vi "TLC Main.vi"() -> ()   [LabVIEW 2009]
doc: "This VI is the Main VI of the Traffic Light Application. The Traffic Light Application is responsible for maintaining traffic at a heavily used 4-way intersection. The intersection includes North, South, East and West bound traffic, with each direction having a left-hand turn lane.\n\nSensors are present at each direction, and the left turn sequence is only inserted if a vehicle is positioned over the left turn lane sensor at the time the left turn sequence should start.\n\nSee the Requirement Document for the detailed pattern of no left-turn and left-turn sequences."
uses:
  controls/tlc_TrafficLightDisplay_cluster.ctl
  controls/tlc_TrafficLightLeftDisplay_cluster.ctl
  modules/controller/tlc_controller_SensorData_cluster.ctl
  controls/tlc_ConsumerDataType_enum.ctl
  controls/tlc_ConsumerCommand_enum.ctl
  modules/error/tlc_error_Command_enum.ctl
  modules/controller/tlc_controller_Command_enum.ctl
panel:
  out "error out":errorcluster
  in  "error in (no error)":errorcluster
  in  "Sensors (type)":T1
  in  "North Sensor":bool
  in  "West Sensor":bool
  in  "East Sensor":bool
  in  "South Sensor":bool
  in  "Stop":bool
  out "West Bound Left":T2
  out "West Bound":T3
  out "North Bound Left":T2
  out "North Bound":T3
  out "East Bound Left":T2
  out "East Bound":T3
  out "South Bound Left":T2
  out "South Bound":T3
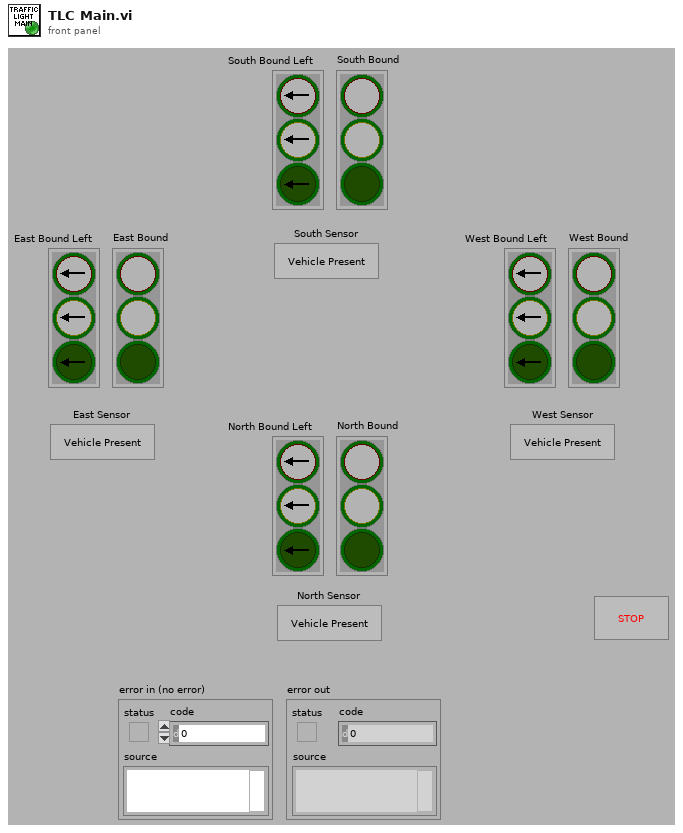
[diagram p1: front panel]
types:
  T1 = typedef "tlc_controller_SensorData_cluster.ctl" = cluster{"South Sensor":bool, "East Sensor":bool, "North Sensor":bool, "West Sensor":bool}
  T2 = typedef "tlc_TrafficLightLeftDisplay_cluster.ctl" = cluster{"Red":bool, "Yellow":bool, "Green":bool}
  T3 = typedef "tlc_TrafficLightDisplay_cluster.ctl" = cluster{"Red":bool, "Yellow":bool, "Green":bool}
  T4 = typedef "tlc_error_Command_enum.ctl" = enum16{"Initialise", "Check Error", "Report Errors"}
  T5 = typedef "tlc_ConsumerDataType_enum.ctl" = cluster{"Command":T6, "Data":variant}
  T6 = typedef "tlc_ConsumerCommand_enum.ctl" = enum16{"Initialise", "Check Controller", "Exit"}
  T7 = typedef "tlc_controller_Command_enum.ctl" = enum16{"Initialise", "Check State", "Next State Logic", "Set Traffic Lights", "Shutdown"}
  T8 = typedef "tlc_controller_TrafficLightsData_cluster.ctl" = cluster{"N/S":T3, "N/S Left":T2, "E/W":T3, "E/W Left":T2}
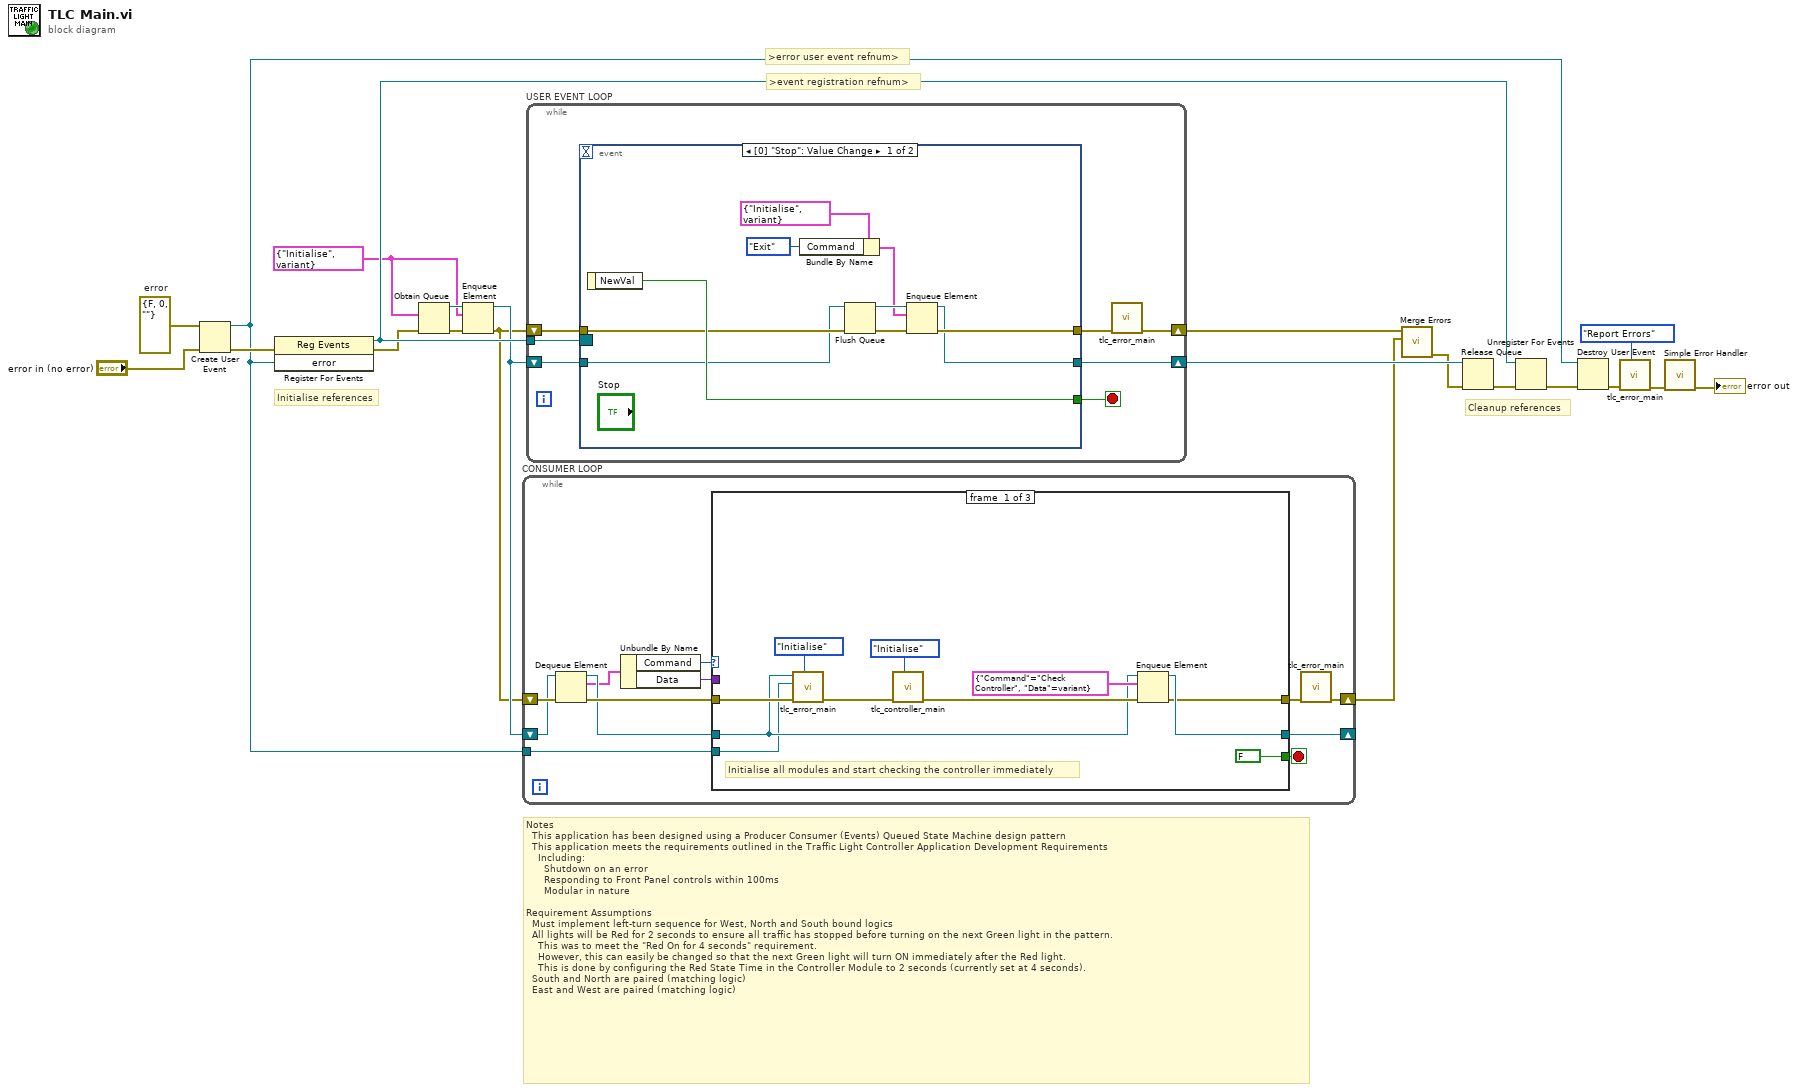
[diagram p0: block diagram]
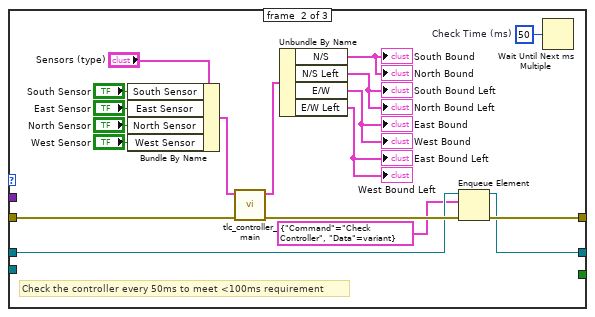
[diagram p2: hidden frame]
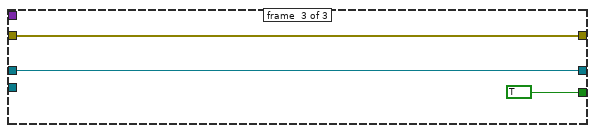
[diagram p3: hidden frame]
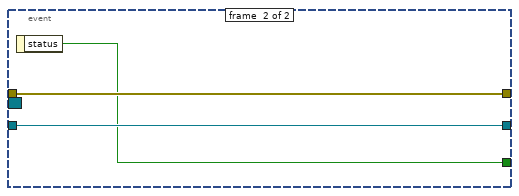
[diagram p4: hidden frame]
diagram:
  w14 = T5 {"Command"=enum."Initialise", "Data"=variant} ("Consumer Data Type")
  w21 = errorcluster {"status"=FALSE, "code"=0, "source"=""}  # error
  # "Notes\n  This application has been designed using a Producer Consumer (Events) Queued State Machine design pattern\n  This application meets the requirements outlined in the Traffic Light Controller Application Development Requirements\n    Including:\n      Shutdown on an error\n      Responding to Front Panel controls within 100ms\n      Modular in nature\n\nRequirement Assumptions\n  Must implement left-turn sequence for West, North and South bound logics\n  All lights will be Red for 2 seconds to ensure all traffic has stopped before turning on the next Green light in the pattern.\n    This was to meet the \"Red On for 4 seconds\" requirement.\n    However, this can easily be changed so that the next Green light will turn ON immediately after the Red light.\n    This is done by configuring the Red State Time in the Controller Module to 2 seconds (currently set at 4 seconds).\n  South and North are paired (matching logic)\n  East and West are paired (matching logic)"
  # "Initialise references"
  # "Cleanup references"
  # ">error user event refnum>"
  # ">event registration refnum>"
  n1 = Create User Event(user event datatype=w21, error in="error in (no error)") -> (user event=w6:refnum<user-event>, error out=w19:errorcluster)
  n2 = register-events(error in=w19, w6) -> (reference out=w18:refnum<event-registration>, error out=w15:errorcluster)  [unwired: 1 in]
  n3 = Obtain Queue(element data type=w14, error in (no error)=w15) -> (queue out=w17:refnum<queue>, error out=w16:errorcluster)  [unwired: 3 in, 1 out]
  n4 = Enqueue Element(queue=w17, element=w14, error in (no error)=w16) -> (queue out=w8:refnum<queue>, error out=w7:errorcluster)  [unwired: 1 in, 1 out]
  n5 = while "CONSUMER LOOP" {
    shift-right: [w33] -> _
    shift-left: w8 -> [w29]
    shift-right: [w23] -> w5
    shift-left: w7 -> [w31]
    tunnel: w6 -> [w32]
    stop <- w24 stop-if-true
    n6 = Dequeue Element(queue=w29, error in (no error)=w31) -> (queue out=w28:refnum<queue>, element=w27:T5, error out=w30:errorcluster)  [unwired: 1 in, 1 out]
    n7 = Unbundle By Name(w27) -> ("Command"=w26:T6, "Data"=w25:variant)
    n8 = case shown="\"Check Controller\"" w26 {
      tunnel: [w34 w50 w65] -> w22
      tunnel: w30 -> [w39 w45 w65]
      tunnel: w28 -> [w37 w49 w64]
      tunnel: [w41 w48 w64] -> w33
      tunnel: w32 -> [w36 _ _]
      tunnel: w25 -> [_ _ _]
      tunnel: [FALSE _ TRUE] -> w24
      frame #0 {
        # "Initialise all modules and start checking the controller immediately"
        n9 = call "tlc_error_main.vi"("Command (Check Error)"=tlc_error_Command_enum."Initialise", "error in (no error)"=w39, "Error User Event Refnum"=w36, "Consumer Queue Refnum"=w37) -> ("error out"=w38:errorcluster)  [unwired: 7 in]
        n10 = call "tlc_controller_main.vi"("Command (Check State)"=tlc_controller_Command_enum."Initialise", "error in (no error)"=w38) -> ("error out"=w40:errorcluster)  [unwired: 8 in, 1 out]
        n11 = Enqueue Element(queue=w37, element=T5 {"Command"=enum."Check Controller", "Data"=variant}, error in (no error)=w40) -> (queue out=w41:refnum<queue>, error out=w34:errorcluster)  [unwired: 1 in, 1 out]
      }
      frame #1 {
        w46 = u32 50  # Check Time (ms)
        # "Check the controller every 50ms to meet <100ms requirement"
        n12 = Bundle By Name(cluster="Sensors (type)", "South Sensor"="South Sensor", "East Sensor"="East Sensor", "North Sensor"="North Sensor", "West Sensor"="West Sensor") -> (w57:T1)
        n13 = call "tlc_controller_main.vi"("error in (no error)"=w45, "Sensors"=w57) -> ("error out"=w51:errorcluster, "Traffic Lights"=w52:T8)  [unwired: 8 in]
        n14 = Unbundle By Name(w52) -> ("N/S"=→"South Bound" →"North Bound":T3, "N/S Left"=→"South Bound Left" →"North Bound Left":T2, "E/W"=→"East Bound" →"West Bound":T3, "E/W Left"=→"East Bound Left" →"West Bound Left":T2)
        n15 = Enqueue Element(queue=w49, element=T5 {"Command"=enum."Check Controller", "Data"=variant}, error in (no error)=w51) -> (queue out=w48:refnum<queue>, error out=w50:errorcluster)  [unwired: 1 in, 1 out]
        n16 = Wait Until Next ms Multiple(millisecond multiple=w46) -> ()  [unwired: 1 out]
      }
      frame #2 {
      }
    }
    n17 = call "tlc_error_main.vi"("error in (no error)"=w22) -> ("error out"=w23:errorcluster)  [unwired: 10 in]
  }
  n18 = while "USER EVENT LOOP" {
    tunnel: w18 -> [w72]
    shift-right: [w67] -> w13
    shift-left: w7 -> [w70]
    shift-right: [w69] -> w12
    shift-left: w8 -> [w71]
    stop <- w68 stop-if-true
    n19 = event shown="[0] \"Stop\": Value Change" {
      selector: w72 -> [_ _]
      dyn-events: _ -> [_ _]
      timeout: _ -> [_ _]
      tunnel: w71 -> [w77 w85]
      tunnel: w70 -> [w81 w84]
      tunnel: [w76 w85] -> w69
      tunnel: [w79 w84] -> w66
      tunnel: [w82 w83] -> w68
      event #0 {
        n20 = event-data() -> ("NewVal"=w82:bool)  [unwired: 1 in]
        n21 = Bundle By Name(cluster=T5 {"Command"=enum."Initialise", "Data"=variant} ("element"), "Command"=tlc_ConsumerCommand_enum."Exit") -> (w74:T5)
        n22 = Flush Queue(queue=w77, error in (no error)=w81) -> (queue out=w78:refnum<queue>, error out=w80:errorcluster)  [unwired: 1 out]
        n23 = Enqueue Element(queue=w78, element=w74, error in (no error)=w80) -> (queue out=w76:refnum<queue>, error out=w79:errorcluster)  [unwired: 1 in, 1 out]
      }
      event #1 {
        n24 = event-data() -> ("status"=w83:bool)  [unwired: 1 in]
      }
    }
    n25 = call "tlc_error_main.vi"("error in (no error)"=w66) -> ("error out"=w67:errorcluster)  [unwired: 10 in]
  }
  n26 = call <vilib>:"Merge Errors.vi"("error in 2 (no error)"=w5, "error in 1 (no error)"=w13) -> ("error out"=w11:errorcluster)  [unwired: 5 in]
  n27 = Release Queue(queue=w12, error in (no error)=w11) -> (error out=w10:errorcluster)  [unwired: 1 in, 2 out]
  n28 = Unregister For Events(event registration refnum=w18, error in=w10) -> (error out=w9:errorcluster)
  n29 = Destroy User Event(user event=w6, error in=w9) -> (error out=w4:errorcluster)
  n30 = call "tlc_error_main.vi"("Command (Check Error)"=tlc_error_Command_enum."Report Errors", "error in (no error)"=w4) -> ("error out"=w2:errorcluster)  [unwired: 9 in]
  n31 = call <vilib>:"Simple Error Handler.vi"("error in (no error)"=w2) -> ("error out"=→"error out":errorcluster)  [unwired: 4 in, 4 out]
